vi "Labspec OpenCom.vi"(8 "error in":errorcluster) -> (0 "error out":errorcluster, 3 "Automation Refnum":refnum<k7>)   [LabVIEW 2014]
panel:
  in  "NFActiveX":refnum<k7>(container)
  # "LICENSED MATERIALS – PROPERTY OF IBM\nCopyright IBM Corp. 2016,\nALL RIGHTS RESERVED"
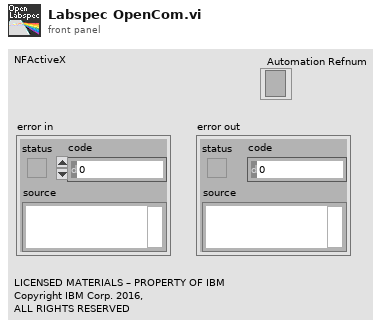
[diagram p1: front panel]
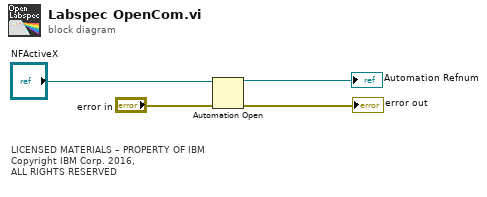
[diagram p0: block diagram]
diagram:
  # "LICENSED MATERIALS – PROPERTY OF IBM\nCopyright IBM Corp. 2016,\nALL RIGHTS RESERVED"
  n1 = Automation Open(error in (no error)="error in", Automation Refnum="NFActiveX") -> (Automation Refnum=→"Automation Refnum":refnum<k7>, error out=→"error out":errorcluster)  [unwired: 1 in, 1 out]
